vi "Arcsec to Rad_ String.vi"(6 "VAR ARCSEC":string) -> (2 "VAR RAD":string, 3 "valid":bool)   [LabVIEW 2018]
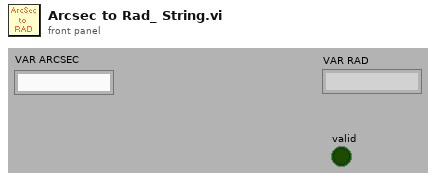
[diagram p1: front panel]
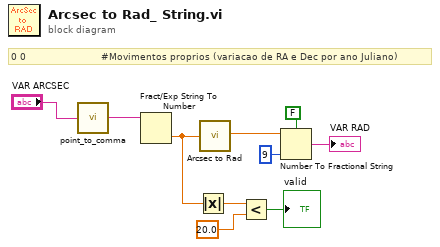
[diagram p0: block diagram]
diagram:
  # "0 0                         #Movimentos proprios (variacao de RA e Dec por ano Juliano)"
  n1 = call "point_to_comma.vi"("Lat_A"="VAR ARCSEC") -> ("Saída"=w9:string)
  n2 = Fract/Exp String To Number(string=w9) -> (number=w4:dbl)  [unwired: 3 in, 1 out]
  n3 = Absolute Value(x=w4) -> (abs(x)=w3:dbl)
  n4 = call "Arcsec to Rad.vi"("Arcsec"=w4) -> ("rad"=w7:dbl)
  n5 = Less?(x=w3, y=20.0) -> (x < y?=→"valid":bool)
  n6 = Number To Fractional String(use system decimal point (T)=FALSE, number=w7, precision (6)=i16 9) -> (F-format string=→"VAR RAD":string)  [unwired: 1 in]
